vi "Cargo Intake Global.vi"() -> ()   [LabVIEW 2018]
panel:
  out "Cargo Sensor":bool
  in  "Cargo Piston":bool
  in  "Calc time diff":bool
  in  "Disable The VI":bool
  out "Cargo Bar Speed":dbl
  in  "Cargo Intake Mode":T1(ring)
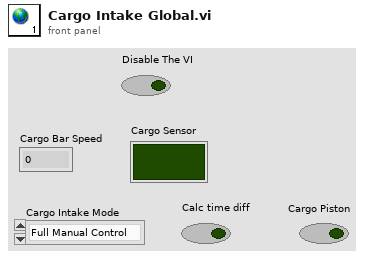
[diagram p1: front panel]
types:
  T1 = enum16{"Full Manual Control", "Manual Control", "Automated Control"}
diagram:
